vi "Read Group Size.vi"(4 "error in (no error)":errorcluster, 6 "Group Number (1)":i32=1 min=1, 7 "VISA resource name":refnum<visa-resource-name>) -> (0 "error out":errorcluster, 2 "Number of axis":i32, 3 "VISA resource name out":refnum<visa-resource-name>)   [LabVIEW 2020, in "Newport ESP301.lvlib"]
doc: "This command is used to read the number of axes assigned to a group."
uses:
  Newport ESP301.lvlib
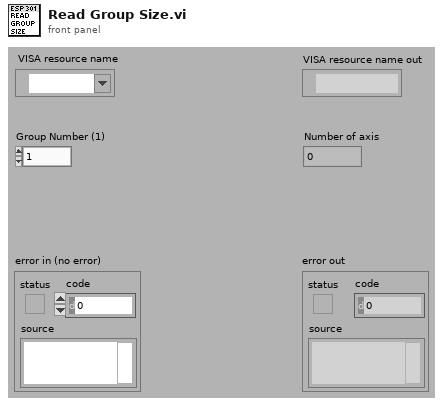
[diagram p1: front panel]
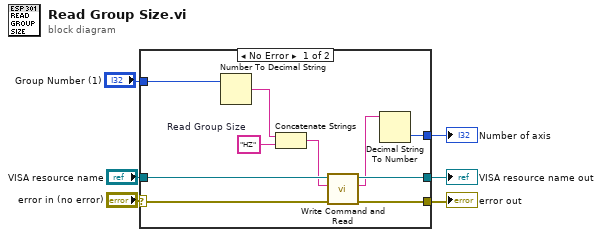
[diagram p0: block diagram]
diagram:
  n1 = case shown="No Error" "error in (no error)" {
    selector: "error in (no error)" -> [w13 w18]
    tunnel: [w15 w18] -> w6
    tunnel: "VISA resource name" -> [w16 w17]
    tunnel: [w14 w17] -> w5
    tunnel: [w11 _] -> w2
    tunnel: "Group Number (1)" -> [w8 _]
    frame No Error {
      w10 = "HZ"  # Read Group Size
      n2 = Number To Decimal String(number=w8) -> (decimal integer string=w9:string)  [unwired: 1 out]
      n3 = Concatenate Strings(w9, w10) -> (w7:string)
      n4 = call "Write Command and Read.vi"("error in (no error)"=w13, "Command"=w7, "VISA resource name"=w16) -> ("error out"=w15:errorcluster, "Returned string"=w12:string, "VISA resource name out"=w14:refnum<visa-resource-name>)  [unwired: 2 in, 2 out]
      n5 = Decimal String To Number(string=w12) -> (number=w11:i32)  [unwired: 2 in, 1 out]
    }
    frame Error {
    }
  }
  "error out" <- w6
  "VISA resource name out" <- w5
  "Number of axis" <- w2
